vi "Add VI to Library.vi"(11 "error in":errorcluster) -> (15 "error out":errorcluster)   [LabVIEW 2021, in "Converter.lvlib"]
uses:
  Converter.lvlib
  Converter Reusables/Converter Reusables.lvlib
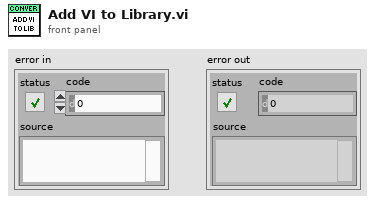
[diagram p1: front panel]
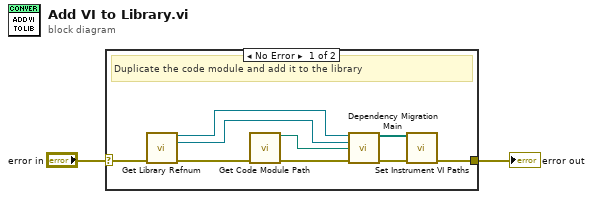
[diagram p0: block diagram]
diagram:
  n1 = case shown="No Error" "error in" {
    selector: "error in" -> [w6 w12]
    tunnel: [w7 w12] -> w1
    frame No Error {
      # "Duplicate the code module and add it to the library"
      n2 = call "Get Library Refnum.vi"("error in"=w6) -> ("library refnum"=w10:refnum<vi>, "project:open"=w11:refnum<vi>, "error out"=w5:errorcluster)  [unwired: 12 in]
      n3 = call "Get Code Module Path.vi"("error in"=w5) -> ("code module out"=w8:path, "error out"=w4:errorcluster)  [unwired: 13 in]
      n4 = call "Dependency Migration Main.vi"("library refnum"=w10, "project:open"=w11, "source module path"=w8, "error in"=w4) -> ("instr containing"=w9:path[], "error out"=w3:errorcluster)  [unwired: 10 in]
      n5 = call "Set Instrument VI Paths.vi"("error in"=w3, "vi paths[]"=w9) -> ("error out"=w7:errorcluster)  [unwired: 9 in]
    }
    frame Error {
    }
  }
  "error out" <- w1
